vi "UpdateOOI List.vi"(0 "Northing":string, 1 "Easting":string, 2 "Type":string, 3 "OOI":string, 4 "Importance":string, 5 "Additional Information":string) -> ()   [LabVIEW 2014]
uses:
  <vilib>/xml/Load XML File.vi
  <vilib>/xml/Close Reference(Node).vi
  <vilib>/xml/NI_XML.lvlib
  <resource>/objmgr/DOMUserDefRef.rc
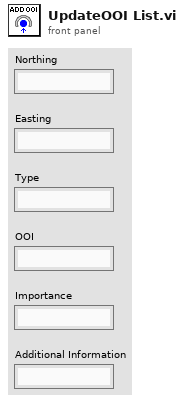
[diagram p1: front panel]
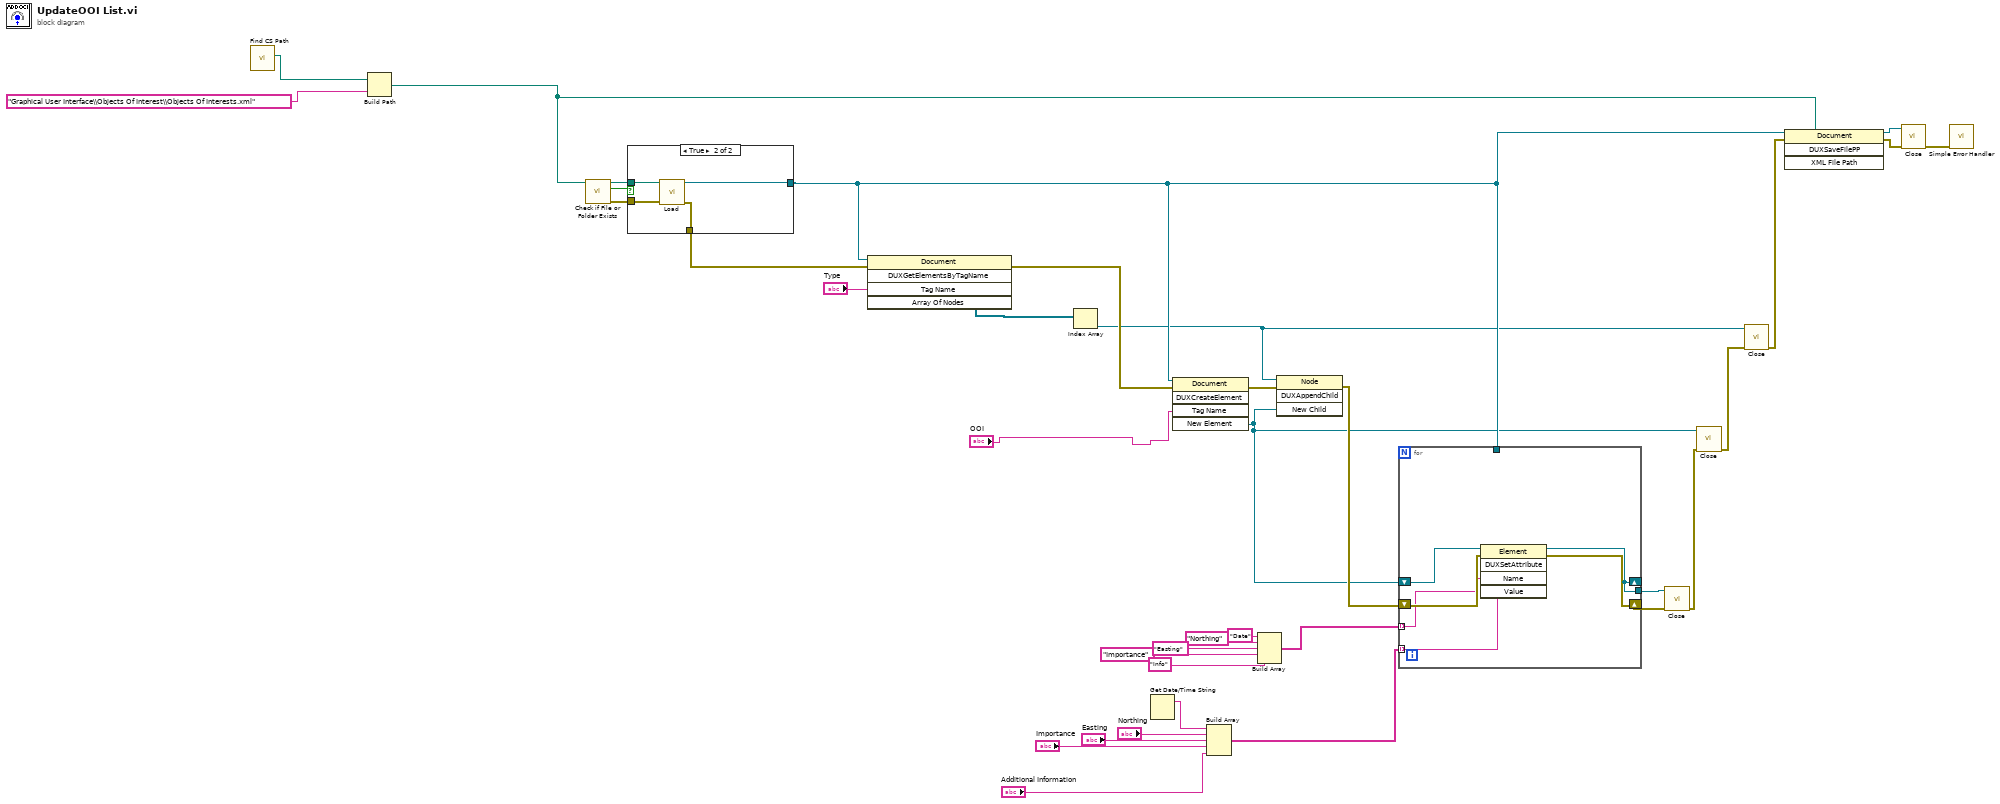
[diagram p0: block diagram]
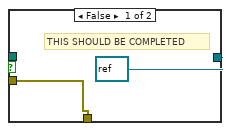
[diagram p2: hidden frame]
diagram:
  n1 = call "Find CS Path.vi"() -> ("path to CS folder"=w4:path)  [unwired: 11 in]
  n2 = Build Path(base path=w4, name or relative path="Graphical User Interface\\Objects Of Interest\\Objects Of Interests.xml") -> (appended path=w2:path)
  n3 = call <vilib>:"Check if File or Folder Exists.vi"("path"=w2) -> ("error out"=w13:errorcluster, "file or folder exists?"=w14:bool, "dup path"=w12:path)  [unwired: 8 in]
  n4 = case shown="True" w14 {
    tunnel: [refnum<k20> refnum ("DOM document out") w42] -> w11
    tunnel: w12 -> [_ w41]
    tunnel: w13 -> [w37 w40]
    tunnel: [w37 w39] -> w18
    frame False {
      # "THIS SHOULD BE COMPLETED"
    }
    frame True {
      n5 = call-poly <vilib>:"Load.vi"("path to XML document"=w41, "error in (no error)"=w40) -> ("DOM document out"=w42:refnum<k20>, "error out"=w39:errorcluster)  [unwired: 11 in, 1 out]
    }
  }
  n6 = invoke class="Document" method="DUXGetElementsByTagName"(reference=w11, error in=w18, "Tag Name"="Type") -> (error out=w16:errorcluster, "Array Of Nodes"=w7:refnum<k20>[])  [unwired: 2 in, 3 out]
  n7 = Index Array(array=w7) -> (element=w6:refnum<k20>)  [unwired: 1 in]
  n8 = Get Date/Time String() -> (date string=w36:string)  [unwired: 3 in, 1 out]
  n9 = invoke class="Document" method="DUXCreateElement"(reference=w11, error in=w16, "Tag Name"="OOI") -> (error out=w19:errorcluster, "New Element"=w10:refnum<k20>)  [unwired: 2 in, 3 out]
  n10 = Build Array(w36, "Northing", "Easting", "Importance", "Additional Information") -> (w8:string[])
  n11 = Build Array("Date" ("element"), "Northing", "Easting", "Importance", "Info") -> (w9:string[])
  n12 = invoke class="Node" method="DUXAppendChild"(reference=w6, error in=w19, "New Child"=w10) -> (error out=w20:errorcluster)  [unwired: 1 in, 3 out]
  n13 = for {
    tunnel: w11 -> [_]
    shift-right: [w44] -> _
    shift-left: w10 -> [w43]
    shift-right: [w45] -> w22
    shift-left: w20 -> [w48]
    tunnel: [w44] -> w5
    tunnel: w9 -> [w47] mode=indexing
    tunnel: w8 -> [w46] mode=indexing
    n14 = invoke class="Element" method="DUXSetAttribute"(reference=w43, error in=w48, "Name"=w47, "Value"=w46) -> (reference out=w44:refnum<k20>, error out=w45:errorcluster)  [unwired: 1 in, 3 out]
  }
  n15 = call-poly <vilib>:"Close.vi"("error in (no error)"=w22, "node"=w5) -> ("error out"=w21:errorcluster)  [unwired: 7 in]
  n16 = call-poly <vilib>:"Close.vi"("error in (no error)"=w21, "node"=w10) -> ("error out"=w15:errorcluster)  [unwired: 7 in]
  n17 = call-poly <vilib>:"Close.vi"("error in (no error)"=w15, "node"=w6) -> ("error out"=w17:errorcluster)  [unwired: 7 in]
  n18 = invoke class="Document" method="DUXSaveFilePP"(reference=w11, error in=w17, "XML File Path"=w2) -> (reference out=w24:refnum<k20>, error out=w25:errorcluster)  [unwired: 1 in, 2 out]
  n19 = call-poly <vilib>:"Close.vi"("error in (no error)"=w25, "node"=w24) -> ("error out"=w23:errorcluster)  [unwired: 7 in]
  n20 = call <vilib>:"Simple Error Handler.vi"("error in (no error)"=w23) -> ()  [unwired: 4 in, 5 out]
